vi "Open_Prefs.vi"(0 "Open Window":bool) -> (1 "Log Files Directory Out":path=path "C:/MOCVD/Log Files", 2 "MOCVD Database File Out":path=path "C:/MOCVD/MOCVD_Growths.accdb", 3 "Use Database Out":bool=TRUE, 4 "Cancelled":bool)   [LabVIEW 2011]
uses:
  low_level_proc/globals.vi
panel:
  in  "Use Database":bool=TRUE
  in  "Cancel":bool
  in  "OK":bool
  in  "MOCVD Database File":path=path "C:/MOCVD/MOCVD_Growths.accdb"
  in  "Log Files Directory":path=path "C:/MOCVD/Log Files"
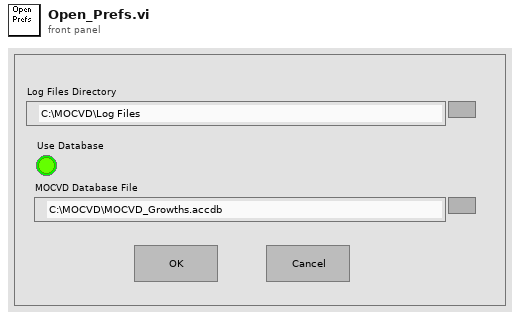
[diagram p1: front panel]
types:
  T1 = enum8{"Enabled", "Disabled", "Disabled and Grayed Out"}
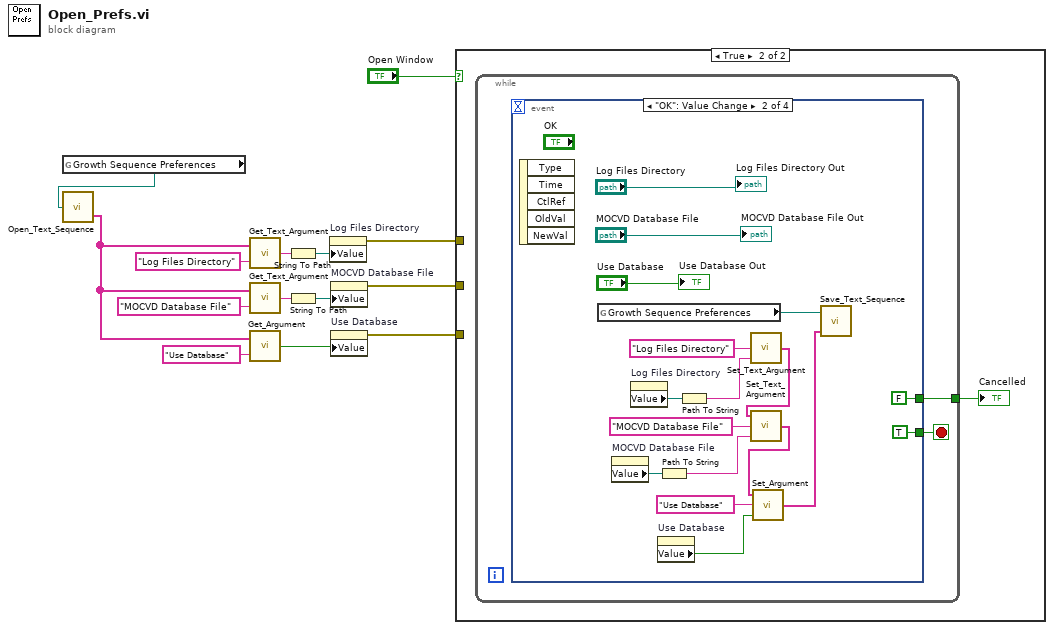
[diagram p0: block diagram]
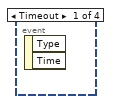
[diagram p3: hidden frame]
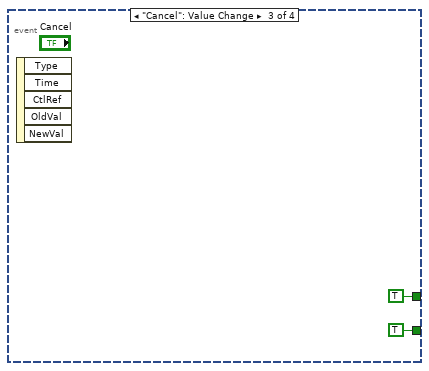
[diagram p4: hidden frame]
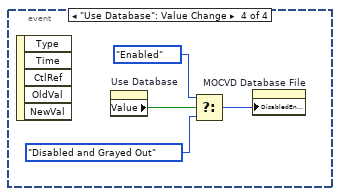
[diagram p5: hidden frame]
diagram:
  n1 = global read "globals.vi" "Growth Sequence Preferences"() -> (w1:path)
  n2 = call "Open_Text_Sequence.vi"("Text File"=w1) -> ("Header"=w7:string[])  [unwired: 1 out]
  n3 = call "Get_Text_Argument.vi"("Argument"="Log Files Directory", "Argument List"=w7) -> ("Text"=w13:string)
  n4 = call "Get_Text_Argument.vi"("Argument"="MOCVD Database File", "Argument List"=w7) -> ("Text"=w9:string)
  n5 = call "Get_Argument.vi"("Argument"="Use Database", "Argument List"=w7) -> ("Enabled"=w5:bool)
  n6 = String To Path(string=w13) -> (path=w12:path)
  n7 = String To Path(string=w9) -> (path=w8:path)
  n8 = property on="Log Files Directory" class="Path"("Value"=w12) -> (error out=w4:errorcluster)  [unwired: 2 in, 1 out]
  n9 = property on="MOCVD Database File" class="Path"("Value"=w8) -> (error out=w3:errorcluster)  [unwired: 2 in, 1 out]
  n10 = property on="Use Database" class="Bool (strict)"("Value"=w5) -> (error out=w2:errorcluster)  [unwired: 2 in, 1 out]
  n11 = case shown="True" "Open Window" {
    tunnel: w4 -> [_ _]
    tunnel: w3 -> [_ _]
    tunnel: w2 -> [_ _]
    frame False {
    }
    frame True {
      n12 = while {
        tunnel: [w17] -> w15
        stop <- w16 stop-if-true
        n13 = event shown="[1] \"OK\": Value Change" {
          selector: _ -> [_ _ _ _]
          dyn-events: _ -> [_ _ _ _]
          timeout: _ -> [_ _ _ _]
          tunnel: [_ FALSE TRUE _] -> w17
          tunnel: [_ TRUE TRUE _] -> w16
          event Timeout {
            n14 = event-data() -> ()  [unwired: 1 in, 2 out]
          }
          event "OK": Value Change {
            n15 = event-data() -> ()  [unwired: 1 in, 5 out]
            n16 = global read "globals.vi" "Growth Sequence Preferences"() -> (w29:path)
            n17 = property on="MOCVD Database File" class="Path"() -> ("Value"=w25:path)  [unwired: 2 in, 2 out]
            n18 = property on="Log Files Directory" class="Path"() -> ("Value"=w23:path)  [unwired: 2 in, 2 out]
            n19 = property on="Use Database" class="Bool (strict)"() -> ("Value"=w27:bool)  [unwired: 2 in, 2 out]
            n20 = Path To String(path=w25) -> (string=w26:string)
            n21 = Path To String(path=w23) -> (string=w24:string)
            n22 = call "Set_Text_Argument.vi"("Text"=w24, "Argument"="Log Files Directory") -> ("Argument List Out"=w19:string[])  [unwired: 1 in]
            n23 = call "Set_Text_Argument.vi"("Text"=w26, "Argument"="MOCVD Database File", "Argument List In"=w19) -> ("Argument List Out"=w21:string[])
            n24 = call "Set_Argument.vi"("Enable"=w27, "Argument"="Use Database", "Argument List In"=w21) -> ("Argument List Out"=w28:string[])
            n25 = call "Save_Text_Sequence.vi"("Header"=w28, "Text File"=w29) -> ()  [unwired: 2 in]
            "Log Files Directory Out" <- "Log Files Directory"
            "MOCVD Database File Out" <- "MOCVD Database File"
            "Use Database Out" <- "Use Database"
          }
          event "Cancel": Value Change {
            n26 = event-data() -> ()  [unwired: 1 in, 5 out]
          }
          event "Use Database": Value Change {
            n27 = event-data() -> ()  [unwired: 1 in, 5 out]
            n28 = property on="Use Database" class="Bool (strict)"() -> ("Value"=w40:bool)  [unwired: 2 in, 2 out]
            n29 = Select(t=T1."Enabled" ("Disabled"), s=w40, f=T1."Disabled and Grayed Out" ("Disabled")) -> (s? t:f=w37:T1)
            n30 = property on="MOCVD Database File" class="Path"("DisabledEnum"=w37) -> ()  [unwired: 2 in, 2 out]
          }
        }
      }
      "Cancelled" <- w15
    }
  }
